vi "viUpdate.vi"(8 "error in (no error)":errorcluster, 11 "OutputPath":path) -> (0 "error out":errorcluster)   [LabVIEW 2018]
doc: "Update the vi from the original one by LabVIEW and SAL \".so\" file."
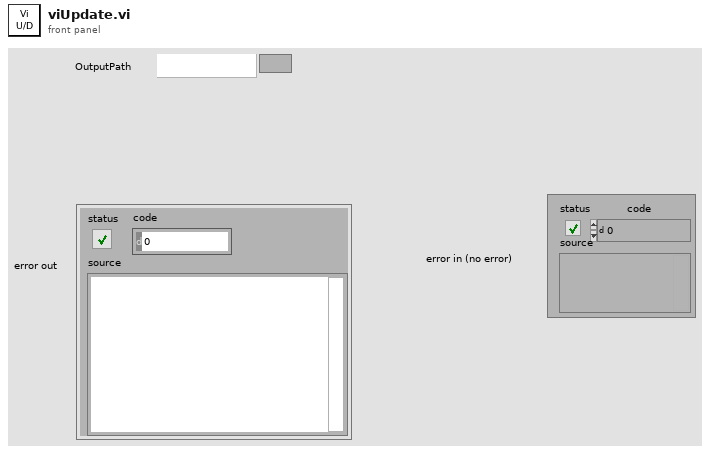
[diagram p1: front panel]
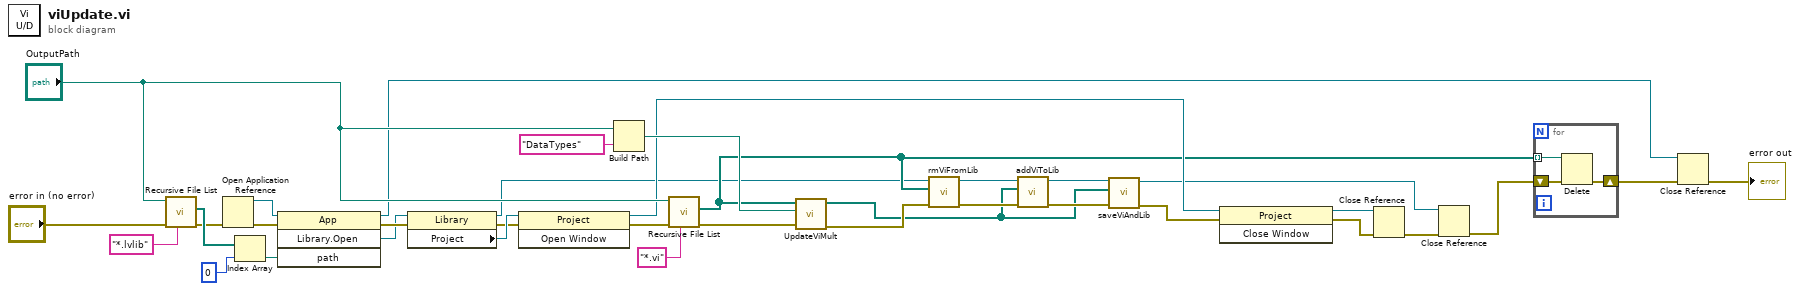
[diagram p0: block diagram]
diagram:
  n1 = call <vilib>:"Recursive File List.vi"("pattern"="*.lvlib", "error in (no error)"="error in (no error)", "Folder Path"="OutputPath") -> ("error out"=w30:errorcluster, "All Files in Dir"=w32:path[])  [unwired: 4 in, 3 out]
  n2 = Open Application Reference(8:w30) -> (0:w28:errorcluster, 3:w29:refnum<vi>)  [unwired: 3 in]
  n3 = Index Array(array=w32, index=0) -> (element=w27:path)
  n4 = invoke class="App" method="Library.Open"(reference=w29, error in=w28, "path"=w27) -> (reference out=w8:refnum<vi>, error out=w25:errorcluster, "Open Library"=w17:refnum<vi>)  [unwired: 1 in, 1 out]
  n5 = property class="Library"(reference=w17, error in=w25) -> (reference out=w11:refnum<vi>, error out=w24:errorcluster, "Project"=w26:refnum<vi>)
  n6 = invoke class="Project" method="Open Window"(reference=w26, error in=w24) -> (reference out=w16:refnum<vi>, error out=w23:errorcluster)  [unwired: 1 in, 1 out]
  n7 = Build Path(base path="OutputPath", name or relative path="DataTypes") -> (appended path=w18:path)
  n8 = call <vilib>:"Recursive File List.vi"("pattern"="*.vi", "error in (no error)"=w23, "Folder Path"="OutputPath") -> ("error out"=w19:errorcluster, "All Files in Dir"=w15:path[])  [unwired: 4 in, 3 out]
  n9 = call "UpdateViMult.vi"("error in (no error)"=w19, "dirOfCtrl"=w18, "arrayOfVi"=w15) -> ("error out"=w13:errorcluster, "arrayOfViRenamed"=w1:path[])  [unwired: 7 in]
  n10 = call "rmViFromLib.vi"("error in (no error)"=w13, "arrayOfVi"=w15, "libRefIn"=w11) -> ("error out"=w12:errorcluster, "libRefInOut"=w14:refnum<vi>)  [unwired: 7 in]
  n11 = call "addViToLib.vi"("error in (no error)"=w12, "arrayOfVi"=w1, "libRefIn"=w14) -> ("error out"=w5:errorcluster, "libRefOut"=w3:refnum<vi>)  [unwired: 7 in]
  n12 = call "saveViAndLib.vi"("error in (no error)"=w5, "arrayOfVi"=w1, "libRefIn"=w3) -> ("error out"=w4:errorcluster, "libRefOut"=w2:refnum<vi>)  [unwired: 7 in]
  n13 = invoke class="Project" method="Close Window"(reference=w16, error in=w4) -> (reference out=w21:refnum<vi>, error out=w22:errorcluster)  [unwired: 1 in, 1 out]
  n14 = Close Reference(reference=w21, error in (no error)=w22) -> (error out=w6:errorcluster)
  n15 = Close Reference(reference=w2, error in (no error)=w6) -> (error out=w7:errorcluster)
  n16 = for {
    shift-right: [w38] -> w10
    shift-left: w7 -> [w39]
    tunnel: w15 -> [w37] mode=indexing
    n17 = Delete(path (use dialog)=w37, error in=w39) -> (error out=w38:errorcluster)  [unwired: 3 in, 2 out]
  }
  n18 = Close Reference(reference=w8, error in (no error)=w10) -> (error out=→"error out":errorcluster)
